vi "Initialize.vi"(0 "VISA resource name":refnum<visa-resource-name>="GPIB0::16::INSTR", 5 "ID Query? (T: Yes)":bool=TRUE, 7 "Reset? (T: Yes)":bool=TRUE, 9 "Serial Configuration":T1={"Baud Rate (9600)"=9600, "Flow Control (1: XON/XOFF)"=1, "Termination Char (0:CR)"=0} {"Termination Char (0:CR)" items=["CR", "LF"]; "Flow Control (1: XON/XOFF)" items=["None", "XON/XOFF", "RTS/CTS (2701 Only)", "XON/XOFF & RTS/CTS (2701 Only)"]; "Baud Rate (9600)" items=["300"=300, "600"=600, "1200"=1200, "2400"=2400, "4800"=4800, "9600"=9600, "19.2k"=19200, "38.4k (2701 Only)"=38400, "57.6k (2701 Only)"=57600, "115.2k (2701 Only)"=115200]}, 11 "error in (no error)":errorcluster) -> (4 "VISA resource name out":refnum<visa-resource-name>, 15 "error out":errorcluster)   [LabVIEW 2013, in "Keithley 27XX.lvlib"]
doc: "This VI opens a VISA session for the VISA resource name specified. You can optionally reset the instrument by setting the front panel reset control. You must run this VI before using any of the instrument driver VIs for this instrument.\n\nNotes:\n\n(1) This instrument driver supports serial communication. If problems are encountered when using serial communication, it is recommended to try using baud rates less than 19,200 and hardware handshaking. \n\n(2) If you do wish to use the serial interface, set the serial settings on the instrument to be the same as the serial settings on the block diagram and in Measurement & Automation Explorer.\n\n(3) This VI sets the instrument to *RST conditions as listed in the manual. This does not include clearing the buffer."
uses:
  <instrlib>/Keithley 27XX/Keithley 27XX.lvlib
panel:
  # "© 2005 National Instruments Corporation.  ALL RIGHTS RESERVED."
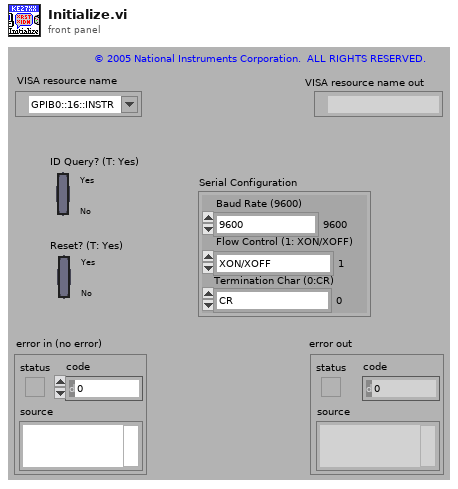
[diagram p1: front panel]
types:
  T1 = cluster{"Baud Rate (9600)":u32, "Flow Control (1: XON/XOFF)":u16, "Termination Char (0:CR)":u16}
  T2 = cluster{"Status":bool, "Code":i32, "Source (VI Name)":string}
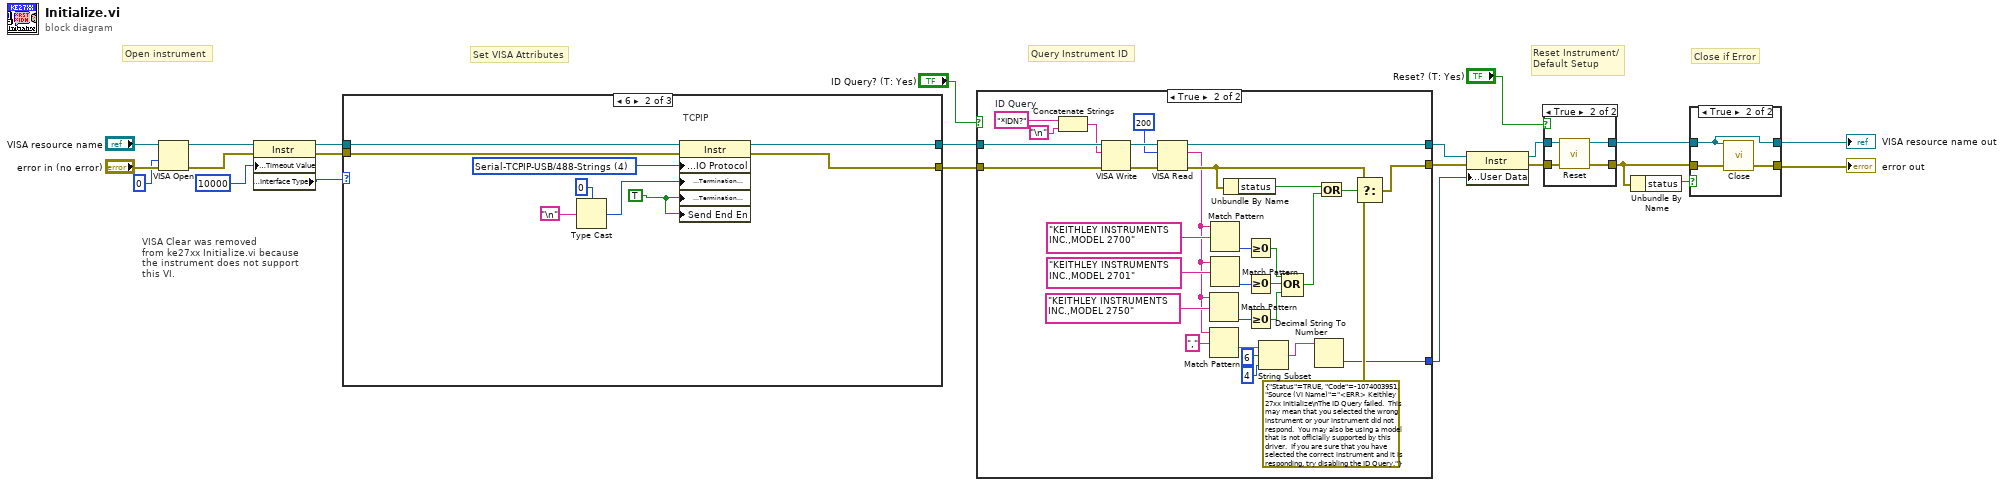
[diagram p0: block diagram]
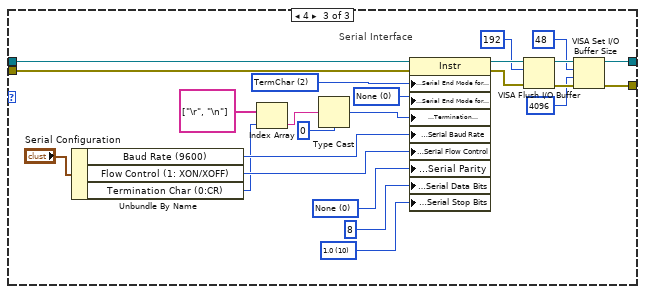
[diagram p3: hidden frame]
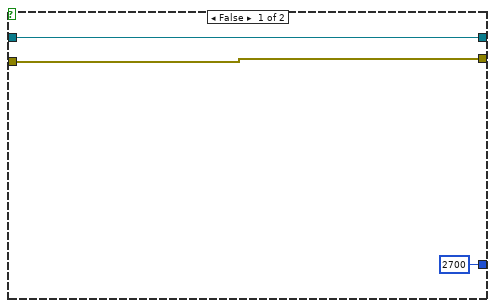
[diagram p6: hidden frame]
diagram:
  # "VISA Clear was removed\nfrom ke27xx Initialize.vi because \nthe instrument does not support\nthis VI."
  # "Set VISA Attributes"
  # "Close if Error"
  # "Query Instrument ID"
  # "Reset Instrument/\nDefault Setup"
  # "Open instrument"
  n1 = VISA Open(access mode=u32 0, error in (no error)="error in (no error)", VISA resource name="VISA resource name") -> (VISA resource name=w1:refnum<visa-resource-name>, error out=w2:errorcluster)  [unwired: 2 in]
  n2 = property class="Instr"(reference=w1, error in=w2, "General Settings:Timeout Value"=u32 10000) -> (reference out=w21:refnum<visa-resource-name>, error out=w22:errorcluster, "Interface Information:Interface Type"=w6:u16)
  n3 = case shown="6" w6 {
    tunnel: [w24 w31 w55] -> w19
    tunnel: [w25 w30 w52] -> w20
    tunnel: w21 -> [w24 w34 w57]
    tunnel: w22 -> [w25 w32 w58]
    frame 1, Default {
      # "GPIB"
    }
    frame 6 {
      w33 = u16 4 items=["Normal"=1, "VXI/FDC"=2, "GPIB/HS488"=3, "Serial-TCPIP-USB/488-Strings"=4, "USBTMC/Vendor-Specific"=5] ("Message Based Settings:IO Protocol")
      w26 = TRUE ("Message Based Settings:Termination Character Enable")
      # "TCPIP"
      n4 = Type Cast(type=u8 0, x="\n") -> (*(type *) &x=w27:u8)
      n5 = property class="Instr"(reference=w34, error in=w32, "Message Based Settings:IO Protocol"=w33, "Message Based Settings:Termination Character"=w27, "Message Based Settings:Termination Character Enable"=w26, "Send End En"=w26) -> (reference out=w31:refnum<visa-resource-name>, error out=w30:errorcluster)
    }
    frame 4 {
      w38 = u16 0 items=["None", "LastBit", "TermChar", "Break"] ("Serial Settings:Serial End Mode for Writes")
      w39 = u16 10 items=["1.0"=10, "1.5"=15, "2.0"=20] ("Serial Settings:Serial Stop Bits")
      w41 = u16 0 items=["None", "Odd", "Even", "Mark", "Space"] ("Serial Settings:Serial Parity")
      w42 = u16 2 items=["None", "LastBit", "TermChar"] ("Serial Settings:Serial End Mode for Reads")
      # "Serial Interface"
      n6 = Unbundle By Name("Serial Configuration") -> ("Baud Rate (9600)"=w44:u32, "Flow Control (1: XON/XOFF)"=w43:u16, "Termination Char (0:CR)"=w35:u16)
      n7 = Index Array(array=string[] ["\r", "\n"], index=w35) -> (element=w37:string)
      n8 = Type Cast(type=u8 0, x=w37) -> (*(type *) &x=w46:u8)
      n9 = property class="Instr"(reference=w57, error in=w58, "Serial Settings:Serial End Mode for Reads"=w42, "Serial Settings:Serial End Mode for Writes"=w38, "Message Based Settings:Termination Character"=w46, "Serial Settings:Serial Baud Rate"=w44, "Serial Settings:Serial Flow Control"=w43, "Serial Settings:Serial Parity"=w41, "Serial Settings:Serial Data Bits"=u16 8, "Serial Settings:Serial Stop Bits"=w39) -> (reference out=w51:refnum<visa-resource-name>, error out=w54:errorcluster)
      n10 = VISA Flush I/O Buffer(VISA resource name=w51, mask (16)=u16 192, error in (no error)=w54) -> (VISA resource name out=w56:refnum<visa-resource-name>, error out=w53:errorcluster)
      n11 = VISA Set I/O Buffer Size(VISA resource name=w56, mask (16)=u16 48, size (4096)=u32 4096 ("size (0)"), error in (no error)=w53) -> (VISA resource name out=w55:refnum<visa-resource-name>, error out=w52:errorcluster)
    }
  }
  n12 = case shown="True" "ID Query? (T: Yes)" {
    tunnel: [w60 w92] -> w8
    tunnel: [w61 w81] -> w11
    tunnel: w19 -> [w61 w84]
    tunnel: w20 -> [w60 w85]
    tunnel: [2700 w65] -> w7
    frame False {
    }
    frame True {
      w64 = "*IDN?"  # ID Query
      n13 = Concatenate Strings(w64, "\n") -> (w62:string)
      n14 = VISA Write(VISA resource name=w84, write buffer=w62, error in (no error)=w85) -> (VISA resource name out=w87:refnum<visa-resource-name>, error out=w86:errorcluster)  [unwired: 1 out]
      n15 = VISA Read(VISA resource name=w87, byte count=u32 200, error in (no error)=w86) -> (VISA resource name out=w81:refnum<visa-resource-name>, read buffer=w78:string, error out=w83:errorcluster)  [unwired: 1 out]
      n16 = Match Pattern(string=w78, regular expression="KEITHLEY INSTRUMENTS INC.,MODEL 2750") -> (offset past match=w75:i32)  [unwired: 1 in, 3 out]
      n17 = Match Pattern(string=w78, regular expression=",") -> (after substring=w69:string)  [unwired: 1 in, 3 out]
      n18 = Match Pattern(string=w78, regular expression="KEITHLEY INSTRUMENTS INC.,MODEL 2700") -> (offset past match=w74:i32)  [unwired: 1 in, 3 out]
      n19 = Match Pattern(string=w78, regular expression="KEITHLEY INSTRUMENTS INC.,MODEL 2701") -> (offset past match=w76:i32)  [unwired: 1 in, 3 out]
      n20 = Unbundle By Name(w83) -> ("status"=w90:bool)
      n21 = Greater Or Equal To 0?(x=w74) -> (x >= 0?=w72:bool)
      n22 = Greater Or Equal To 0?(x=w76) -> (x >= 0?=w73:bool)
      n23 = Greater Or Equal To 0?(x=w75) -> (x >= 0?=w71:bool)
      n24 = String Subset(string=w69, offset (0)=6, length (rest)=4 ("length (rest)")) -> (substring=w66:string)
      n25 = Compound Arithmetic op=OR(w72, w73, w71) -> (w70:bool)
      n26 = Decimal String To Number(string=w66) -> (number=w65:i32)  [unwired: 2 in, 1 out]
      n27 = Or(x=w90, y=w70) -> (x .or. y?=w91:bool)
      n28 = Select(t=w83, s=w91, f=T2 {"Status"=TRUE, "Code"=-1074003951, "Source (VI Name)"="<ERR> Keithley 27xx Initialize\nThe ID Query failed.  This may mean that you selected the wrong instrument or your instrument did not respond.  You may also be using a model that is not officially supported by this driver.  If you are sure that you have selected the correct instrument and it is responding, try disabling the ID Query."}) -> (s? t:f=w92:T2)
    }
  }
  n29 = property on="Property Node" class="Instr"(reference=w11, error in=w8, "General Settings:User Data"=w7) -> (reference out=w10:refnum<visa-resource-name>, error out=w9:errorcluster)
  n30 = case shown="True" "Reset? (T: Yes)" {
    tunnel: w9 -> [w93 w97]
    tunnel: [w93 w96] -> w12
    tunnel: w10 -> [w94 w98]
    tunnel: [w94 w95] -> w13
    frame False {
    }
    frame True {
      n31 = call <instrlib>:"Reset.vi"("VISA resource name"=w98, "error in (no error)"=w97) -> ("VISA resource name out"=w95:refnum<visa-resource-name>, "error out"=w96:errorcluster)  [unwired: 12 in]
    }
  }
  n32 = Unbundle By Name(w12) -> ("status"=w23:bool)
  n33 = case shown="True" w23 {
    tunnel: w13 -> [w100 w101]
    tunnel: [w100 w101] -> w5
    tunnel: [w99 w102] -> w4
    tunnel: w12 -> [w99 w103]
    frame False {
    }
    frame True {
      n34 = call <instrlib>:"Close.vi"("VISA resource name"=w101, "error in (no error)"=w103) -> ("error out"=w102:errorcluster)  [unwired: 13 in]
    }
  }
  "VISA resource name out" <- w5
  "error out" <- w4
